vi "Test New Image.vi"(8 "error in (no error)":errorcluster, 11 "Test Case In":refnum<class "Image.lvclass">) -> (0 "error out":errorcluster, 3 "Test Case Out":refnum<class "Image.lvclass">)   [LabVIEW 2020, in "g_ar_toolkit.test.lvlib" / "Image.lvclass"]
uses:
  Image.lvclass
  C:/Program Files (x86)/National Instruments/LabVIEW 2020/vi.lib/Astemes/LUnit/Test Case.lvclass
  g_ar_toolkit.common/Image Size (Integer).ctl
  <vilib>/Astemes/LUnit/Test Case.lvclass/Test Case.ctl
  g_ar_toolkit.image/ARGB Colour.ctl
  0bcaab8e-db39-49f4-b03c-e96854e28b99.vi
  g_ar_toolkit.image/New Image (ARGB).vi
  4247fbd1-0910-49f6-b629-9f858556f783.vi
  g_ar_toolkit.image/New Image (Greyscale).vi
  ec21ac67-ee19-4f7a-8949-2d8c4815d422.vi
  ef19801d-c7eb-448b-804c-03b939946be6.vi
  a2513b5f-71c0-4474-9565-80dd8f5665c2.vi
  g_ar_toolkit.image/New Image (ARGB Array).vi
  a0ca83e2-f906-46f0-9900-73016ca927a2.vi
  2c97c103-d6e4-4ea7-8e02-490b8170dd99.vi
  g_ar_toolkit.image/New Image (Greyscale Array).vi
  9bbea696-5130-4afb-936d-006bbeed6fe9.vi
  4769743d-9c77-4430-a324-349858fd9cd5.vi
  8addd5ea-cbc8-4cc4-a329-325e9d80df7e.vi
  g_ar_toolkit.image/New Image (ARGB).vi/3321fa97-f432-4e1e-8db9-a0df79aed21b.vi
  <vilib>/Astemes/LUnit/Append Pass Result.vi
  <vilib>/Astemes/LUnit/Append Fail Result.vi
  <vilib>/Astemes/LUnit/Describe Comparison.vi
  4247fbd1-0910-49f6-b629-9f858556f783.vi/9c5d11cd-9439-4240-a1ee-d9baace9c924.vi
  g_ar_toolkit.image/New Image (Greyscale).vi/6598b9e0-8a08-46f5-91fd-ca1b87217137.vi
  ec21ac67-ee19-4f7a-8949-2d8c4815d422.vi/9c5d11cd-9439-4240-a1ee-d9baace9c924.vi
  ef19801d-c7eb-448b-804c-03b939946be6.vi/9c5d11cd-9439-4240-a1ee-d9baace9c924.vi
  a2513b5f-71c0-4474-9565-80dd8f5665c2.vi/9c5d11cd-9439-4240-a1ee-d9baace9c924.vi
  a0ca83e2-f906-46f0-9900-73016ca927a2.vi/9c5d11cd-9439-4240-a1ee-d9baace9c924.vi
  2c97c103-d6e4-4ea7-8e02-490b8170dd99.vi/9c5d11cd-9439-4240-a1ee-d9baace9c924.vi
  9bbea696-5130-4afb-936d-006bbeed6fe9.vi/9c5d11cd-9439-4240-a1ee-d9baace9c924.vi
  4769743d-9c77-4430-a324-349858fd9cd5.vi/9c5d11cd-9439-4240-a1ee-d9baace9c924.vi
  8addd5ea-cbc8-4cc4-a329-325e9d80df7e.vi/9c5d11cd-9439-4240-a1ee-d9baace9c924.vi
  <vilib>/Astemes/LUnit/Run In UI.vi
  <vilib>/Utility/error.llb/Clear Errors.vi
  g_ar_toolkit.common/Module Path.vi
  <vilib>/Utility/error.llb/Error Cluster From Error Code.vi
  <vilib>/Astemes/LUnit/Describe Variant.vi
  Image.lvclass/Image.ctl
  g_ar_toolkit.image/g_ar_toolkit.image.lvlib
  g_ar_toolkit.common/g_ar_toolkit.common.lvlib
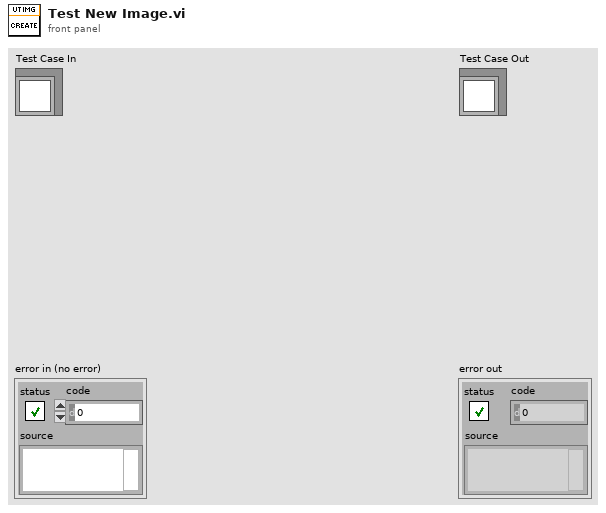
[diagram p1: front panel]
types:
  T1 = enum16{"ARGB empty", "Greyscale empty", "ARGB with size", "Greyscale with size", "ARGB from Array", "ARGB from Array force Alpha", "Greyscale from Array", "ARGB from Array Empty", "Greyscale from Array Empty"}
  T2 = typedef "g_ar_toolkit.common.lvlib/Image Size (Integer).ctl" = cluster{"Width":u16, "Height":u16}
  T3 = enum16{"ARGB empty", "Greyscale empty", "ARGB with size", "Greyscale with size", "ARGB from Array", "ARGB from Array force Alpha", "Greyscale from Array", "ARGB from Array Empty", "Greyscale from Array Empty"}[]
  T4 = typedef "g_ar_toolkit.image.lvlib/ARGB Colour.ctl" = cluster{"Alpha":u8, "RGB":u32}
  T5 = typedef "g_ar_toolkit.image.lvlib/ARGB Image.ctl" = refnum<data-value>
  T6 = typedef "g_ar_toolkit.image.lvlib/Greyscale Image.ctl" = refnum<data-value>
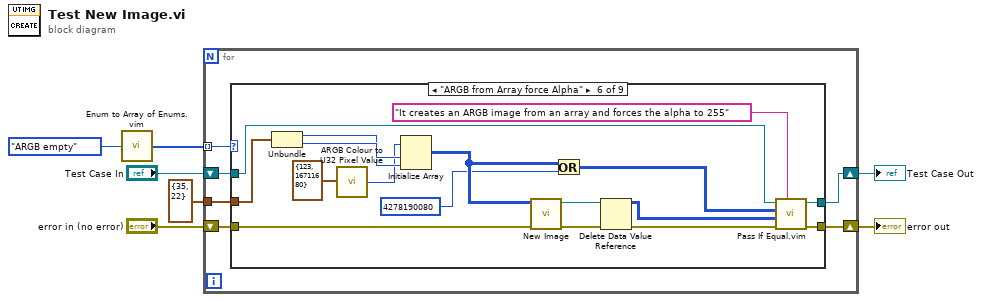
[diagram p0: block diagram]
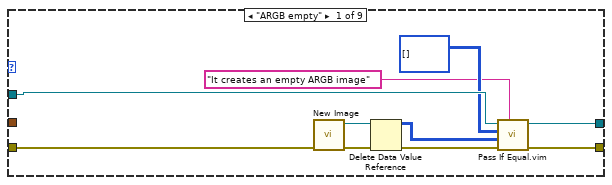
[diagram p2: hidden frame]
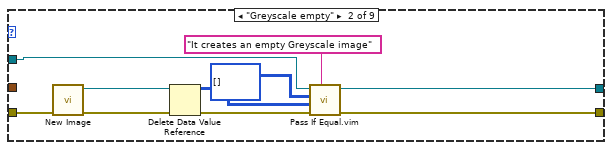
[diagram p3: hidden frame]
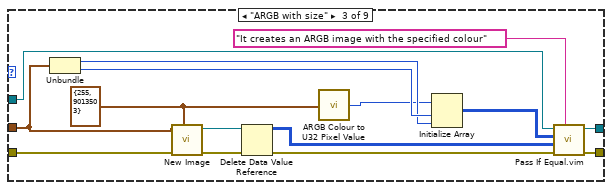
[diagram p4: hidden frame]
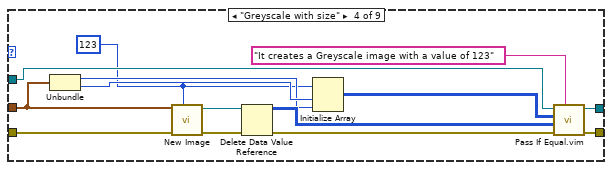
[diagram p5: hidden frame]
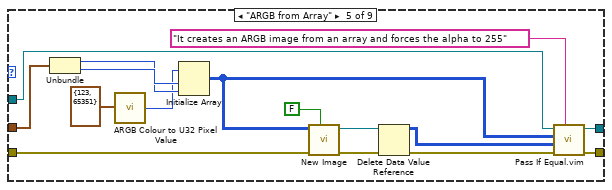
[diagram p6: hidden frame]
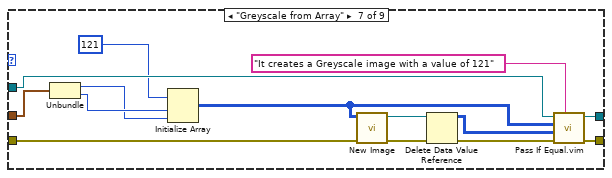
[diagram p7: hidden frame]
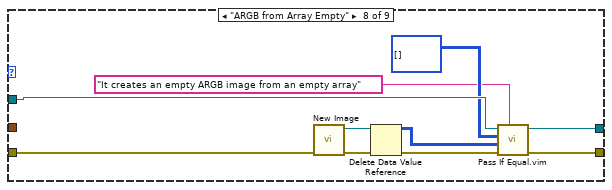
[diagram p8: hidden frame]
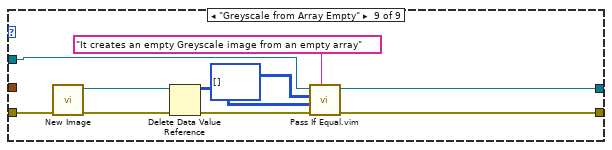
[diagram p9: hidden frame]
diagram:
  n1 = call "Enum to Array of Enums.vim"("enum"=T1."ARGB empty") -> ("array of enums"=w2:T3)
  n2 = for {
    shift-right: [w10] -> w6
    shift-left: "Test Case In" -> [w13]
    shift-right: [w9] -> w4
    shift-left: "error in (no error)" -> [w12]
    tunnel: w2 -> [w11] mode=indexing
    tunnel: T2 {"Width"=35, "Height"=22} ("Preallocated Image Size (Default: 0,0)") -> [w8]
    n3 = case shown="\"ARGB from Array force Alpha\"" w11 {
      tunnel: w13 -> [w17 w30 w42 w56 w72 w89 w103 w113 w126]
      tunnel: w12 -> [w23 w33 w48 w62 w78 w95 w109 w119 w129]
      tunnel: [w18 w29 w43 w57 w73 w90 w104 w114 w125] -> w10
      tunnel: [w19 w27 w44 w58 w74 w91 w105 w115 w123] -> w9
      tunnel: w8 -> [_ _ w34 w49 w67 w84 w98 _ _]
      frame "ARGB empty" {
        n4 = call-poly "New Image.vi"("error in (no error)"=w23) -> ("error out"=w22:errorcluster, "New ARGB Image"=w21:T5)  [unwired: 9 in]
        n5 = Delete Data Value Reference(data value reference=w21, error in=w22) -> (data value=w16:u32[][], error out=w20:errorcluster)
        n6 = call "Pass If Equal.vim"("Description"="It creates an empty ARGB image", "error in (no error)"=w20, "Actual"=w16, "Expected"=u32[][] [] ("data value"), "LUnit Test Case In"=w17) -> ("error out"=w19:errorcluster, "LUnit Test Case Out"=w18:refnum<class "Image.lvclass">)  [unwired: 5 in]
      }
      frame "Greyscale empty" {
        n7 = call-poly "New Image.vi"("error in (no error)"=w33) -> ("error out"=w32:errorcluster, "New Greyscale Image"=w31:T6)  [unwired: 9 in]
        n8 = Delete Data Value Reference(data value reference=w31, error in=w32) -> (data value=w25:u8[][], error out=w28:errorcluster)
        n9 = call "Pass If Equal.vim"("Description"="It creates an empty Greyscale image", "error in (no error)"=w28, "Actual"=w25, "Expected"=u8[][] [] ("data value"), "LUnit Test Case In"=w30) -> ("error out"=w27:errorcluster, "LUnit Test Case Out"=w29:refnum<class "Image.lvclass">)  [unwired: 5 in]
      }
      frame "ARGB with size" {
        w36 = T4 {"Alpha"=255, "RGB"=9013503} ("Colour (Default: Black)")
        n10 = Unbundle(w34) -> ("Width"=w38:u16, "Height"=w39:u16)
        n11 = call-poly "New Image.vi"("Colour (Default: Black)"=w36, "error in (no error)"=w48, "Preallocated Image Size (Default: 0,0)"=w34) -> ("error out"=w47:errorcluster, "New ARGB Image"=w46:T5)  [unwired: 7 in]
        n12 = Delete Data Value Reference(data value reference=w46, error in=w47) -> (data value=w41:u32[][], error out=w45:errorcluster)
        n13 = call "ARGB Colour to U32 Pixel Value.vi"("ARGB Colour"=w36) -> ("U32 Colour"=w35:u32)
        n14 = Initialize Array(w35, w39, w38) -> (w37:u32[][])
        n15 = call "Pass If Equal.vim"("Description"="It creates an ARGB image with the specified colour", "error in (no error)"=w45, "Actual"=w41, "Expected"=w37, "LUnit Test Case In"=w42) -> ("error out"=w44:errorcluster, "LUnit Test Case Out"=w43:refnum<class "Image.lvclass">)  [unwired: 5 in]
      }
      frame "Greyscale with size" {
        w50 = u8 123 ("Value (Default: 0)")
        n16 = Unbundle(w49) -> ("Width"=w52:u16, "Height"=w53:u16)
        n17 = call-poly "New Image.vi"("Value (Default: 0)"=w50, "error in (no error)"=w62, "Preallocated Image Size (Default 0,0)"=w49) -> ("error out"=w61:errorcluster, "New Greyscale Image"=w60:T6)  [unwired: 7 in]
        n18 = Delete Data Value Reference(data value reference=w60, error in=w61) -> (data value=w55:u8[][], error out=w59:errorcluster)
        n19 = Initialize Array(w50, w53, w52) -> (w51:u8[][])
        n20 = call "Pass If Equal.vim"("Description"="It creates a Greyscale image with a value of 123", "error in (no error)"=w59, "Actual"=w55, "Expected"=w51, "LUnit Test Case In"=w56) -> ("error out"=w58:errorcluster, "LUnit Test Case Out"=w57:refnum<class "Image.lvclass">)  [unwired: 5 in]
      }
      frame "ARGB from Array" {
        n21 = Unbundle(w67) -> ("Width"=w68:u16, "Height"=w69:u16)
        n22 = call "ARGB Colour to U32 Pixel Value.vi"("ARGB Colour"=T4 {"Alpha"=123, "RGB"=65351} ("Colour (Default: Black)")) -> ("U32 Colour"=w65:u32)
        n23 = Initialize Array(w65, w69, w68) -> (w64:u32[][])
        n24 = call-poly "New Image.vi"("Set Alpha Values to 255 (Default: True)"=FALSE, "error in (no error)"=w78, "U32 ARBG Data  (Default: Empty)"=w64) -> ("error out"=w77:errorcluster, "New ARGB Image"=w76:T5)  [unwired: 7 in]
        n25 = Delete Data Value Reference(data value reference=w76, error in=w77) -> (data value=w71:u32[][], error out=w75:errorcluster)
        n26 = call "Pass If Equal.vim"("Description"="It creates an ARGB image from an array and forces the alpha to 255", "error in (no error)"=w75, "Actual"=w71, "Expected"=w64, "LUnit Test Case In"=w72) -> ("error out"=w74:errorcluster, "LUnit Test Case Out"=w73:refnum<class "Image.lvclass">)  [unwired: 5 in]
      }
      frame "ARGB from Array force Alpha" {
        n27 = Unbundle(w84) -> ("Width"=w85:u16, "Height"=w86:u16)
        n28 = call "ARGB Colour to U32 Pixel Value.vi"("ARGB Colour"=T4 {"Alpha"=123, "RGB"=16711680} ("Colour (Default: Black)")) -> ("U32 Colour"=w82:u32)
        n29 = Initialize Array(w82, w86, w85) -> (w81:u32[][])
        n30 = call-poly "New Image.vi"("error in (no error)"=w95, "U32 ARBG Data  (Default: Empty)"=w81) -> ("error out"=w94:errorcluster, "New ARGB Image"=w93:T5)  [unwired: 8 in]
        n31 = Or(x=w81, y=u32 4278190080 ("U32 Colour")) -> (x .or. y?=w80:u32[][])
        n32 = Delete Data Value Reference(data value reference=w93, error in=w94) -> (data value=w88:u32[][], error out=w92:errorcluster)
        n33 = call "Pass If Equal.vim"("Description"="It creates an ARGB image from an array and forces the alpha to 255", "error in (no error)"=w92, "Actual"=w88, "Expected"=w80, "LUnit Test Case In"=w89) -> ("error out"=w91:errorcluster, "LUnit Test Case Out"=w90:refnum<class "Image.lvclass">)  [unwired: 5 in]
      }
      frame "Greyscale from Array" {
        n34 = Unbundle(w98) -> ("Width"=w99:u16, "Height"=w100:u16)
        n35 = Initialize Array(u8 121 ("Value (Default: 0)"), w100, w99) -> (w96:u8[][])
        n36 = call-poly "New Image.vi"("error in (no error)"=w109, "Greyscale Pixels (Default: Empty)"=w96) -> ("error out"=w108:errorcluster, "Greyscale Image"=w107:T6)  [unwired: 8 in]
        n37 = Delete Data Value Reference(data value reference=w107, error in=w108) -> (data value=w102:u8[][], error out=w106:errorcluster)
        n38 = call "Pass If Equal.vim"("Description"="It creates a Greyscale image with a value of 121", "error in (no error)"=w106, "Actual"=w102, "Expected"=w96, "LUnit Test Case In"=w103) -> ("error out"=w105:errorcluster, "LUnit Test Case Out"=w104:refnum<class "Image.lvclass">)  [unwired: 5 in]
      }
      frame "ARGB from Array Empty" {
        n39 = call-poly "New Image.vi"("error in (no error)"=w119) -> ("error out"=w118:errorcluster, "New ARGB Image"=w117:T5)  [unwired: 9 in]
        n40 = Delete Data Value Reference(data value reference=w117, error in=w118) -> (data value=w112:u32[][], error out=w116:errorcluster)
        n41 = call "Pass If Equal.vim"("Description"="It creates an empty ARGB image from an empty array", "error in (no error)"=w116, "Actual"=w112, "Expected"=u32[][] [] ("data value"), "LUnit Test Case In"=w113) -> ("error out"=w115:errorcluster, "LUnit Test Case Out"=w114:refnum<class "Image.lvclass">)  [unwired: 5 in]
      }
      frame "Greyscale from Array Empty" {
        n42 = call-poly "New Image.vi"("error in (no error)"=w129) -> ("error out"=w128:errorcluster, "Greyscale Image"=w127:T6)  [unwired: 9 in]
        n43 = Delete Data Value Reference(data value reference=w127, error in=w128) -> (data value=w121:u8[][], error out=w124:errorcluster)
        n44 = call "Pass If Equal.vim"("Description"="It creates an empty Greyscale image from an empty array", "error in (no error)"=w124, "Actual"=w121, "Expected"=u8[][] [] ("data value"), "LUnit Test Case In"=w126) -> ("error out"=w123:errorcluster, "LUnit Test Case Out"=w125:refnum<class "Image.lvclass">)  [unwired: 5 in]
      }
    }
  }
  "error out" <- w4
  "Test Case Out" <- w6
